vi "Report Event.vi"(7 "Level (Info)":T1=enum."Info", 8 "error in (no error)":errorcluster, 9 "Message":string, 11 "Task in":refnum<class "Task.lvclass">) -> (0 "error out":errorcluster, 3 "Task out":refnum<class "Task.lvclass">)   [LabVIEW 2020, in "Volatus.lvlib" / "Task.lvclass"]
uses:
  Task.lvclass
  Event Level.ctl
  Task.lvclass/Task.ctl
  Event API/EventAPI.lvclass/EventAPI.ctl
  EventHandler Messages/Handle Event Msg/Handle Event Msg.lvclass/Handle Event Msg.ctl
  <vilib>/ActorFramework/Message Enqueuer/Message Enqueuer.lvclass/Message Enqueuer.ctl
  EventHandler Messages/Handle Event Msg/Send Handle Event.vi
  <vilib>/ActorFramework/Message Enqueuer/Enqueue.vi
  EventHandler Messages/Handle Event Msg/Handle Event Msg.lvclass
  C:/Program Files (x86)/National Instruments/LabVIEW 2020/vi.lib/ActorFramework/Message/Message.lvclass
  <vilib>/ActorFramework/Message Priority Queue/Priority Enqueue.vi
  Event API/EventAPI.lvclass
  Volatus.lvlib
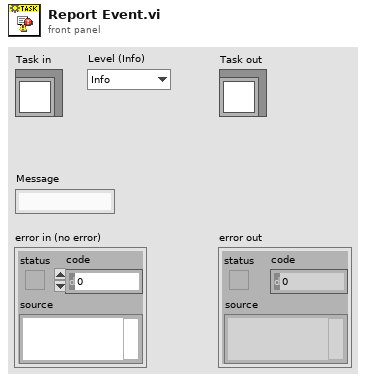
[diagram p1: front panel]
types:
  T1 = typedef "Volatus.lvlib/Event Level.ctl" = enum16{"Debug", "Info", "Warning", "Error"}
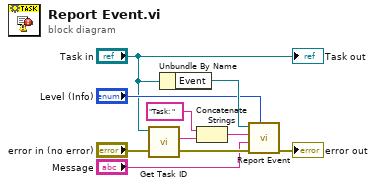
[diagram p0: block diagram]
diagram:
  n1 = call "Get Task ID.vi"("Task in"="Task in") -> ("Task ID"=w3:string)  [unwired: 9 in, 1 out]
  n2 = Unbundle By Name("Task in") -> ("Event"=w9:refnum<class "EventAPI.lvclass">)
  n3 = Concatenate Strings("Task: ", w3) -> (w1:string)
  n4 = call "Report Event.vi"("Level (Info)"="Level (Info)", "error in (no error)"="error in (no error)", "Message"="Message", "Context"=w1, "Event API in"=w9) -> ("error out"=→"error out":errorcluster)  [unwired: 5 in, 1 out]
  "Task out" <- "Task in"
